vi "ParaSet_1.vi"(11 "Controls":T1) -> (3 "String":string)   [LabVIEW 2014, in "Programing Logic.lvclass"]
uses:
  Programming Logic/Programing Logic.lvclass
  Controls/ParaSet.ctl
  Controls/Control Library.lvlib
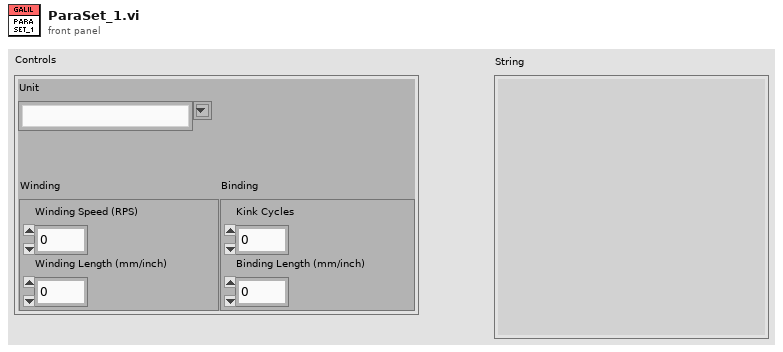
[diagram p1: front panel]
types:
  T1 = typedef "Control Library.lvlib/ParaSet.ctl" = cluster{"Unit":string, "Winding":cluster{"Winding Speed (RPS)":dbl, "Winding Length (mm/inch)":dbl}, "Binding":cluster{"Kink Cycles":dbl, "Binding Length (mm/inch)":dbl}}
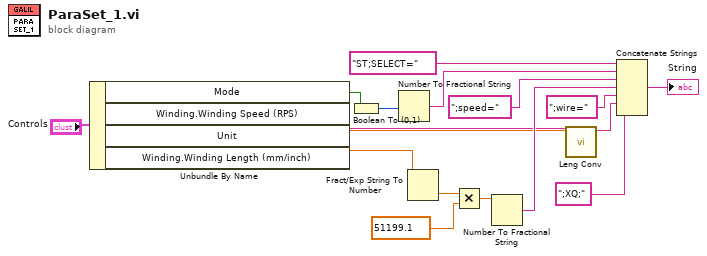
[diagram p0: block diagram]
diagram:
  n1 = Unbundle By Name("Controls") -> ("Mode"=w4:bool, "Winding.Winding Speed (RPS)"=w2:dbl, "Unit"=w1:string, "Winding.Winding Length (mm/inch)"=w3:dbl)
  n2 = Boolean To (0,1)(Boolean=w4) -> (0, 1=w8:i16)
  n3 = Number To Fractional String(number=w8) -> (F-format string=w7:string)  [unwired: 3 in]
  n4 = Fract/Exp String To Number(string=w3) -> (number=w12:dbl)  [unwired: 3 in, 1 out]
  n5 = Multiply(x=w12, y=51199.1) -> (x*y=w14:dbl)
  n6 = Number To Fractional String(number=w14) -> (F-format string=w15:string)  [unwired: 3 in]
  n7 = call "Leng Conv.vi"("Unit"=w1, "Winding Length"=w2) -> ("String"=w6:string)  [unwired: 9 in]
  n8 = Concatenate Strings("ST;SELECT=" ("string"), w7, ";speed=" ("string"), w15, ";wire=" ("string"), w6, ";XQ;" ("string")) -> (→"String":string)
